vi "Array Max N points.vi"(10 "N":i32, 11 "U8 Array in":u8[](array[numeric])) -> (1 "N Greatest Values":u8[](array[numeric]), 3 "N greatest indicies":i32[](array[numeric]))   [LabVIEW 2013]
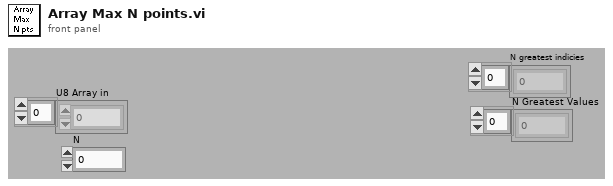
[diagram p1: front panel]
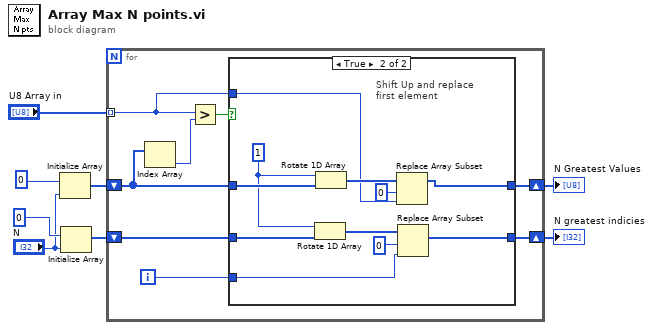
[diagram p0: block diagram]
diagram:
  n1 = Initialize Array(u8 0, "N") -> (w3:u8[])
  n2 = Initialize Array(0 ("N"), "N") -> (w6:i32[])
  n3 = for {
    tunnel: "U8 Array in" -> [w10] mode=indexing
    shift-right: [w13] -> w7
    shift-left: w6 -> [w14]
    shift-right: [w11] -> w5
    shift-left: w3 -> [w12]
    i -> [w15]
    n4 = Index Array(array=w12) -> (element=w16:u8)  [unwired: 1 in]
    n5 = Greater?(x=w10, y=w16) -> (0:w9:bool)
    n6 = case shown="True" w9 {
      tunnel: w15 -> [_ w21]
      tunnel: w14 -> [w18 w28]
      tunnel: [w18 w22] -> w13
      tunnel: w12 -> [w17 w29]
      tunnel: [w17 w25] -> w11
      tunnel: w10 -> [_ w20]
      frame False {
      }
      frame True {
        w19 = 1 ("n")
        # "Shift Up and replace\nfirst element"
        n7 = Rotate 1D Array(1:w28, 2:w19) -> (0:w24:i32[])
        n8 = Rotate 1D Array(1:w29, 2:w19) -> (0:w27:u8[])
        n9 = Replace Array Subset(array=w27, new element=w20, index=0) -> (w25:u8[])
        n10 = Replace Array Subset(array=w24, new element=w21, index=0) -> (w22:i32[])
      }
    }
  }
  "N greatest indicies" <- w7
  "N Greatest Values" <- w5
